vi "Auton File Loader.vi"() -> ()   [LabVIEW 2017]
uses:
  Common Code/Auton File Lists.ctl
  Robot Global Data.vi
panel:
  in  "Auton File Lists":T1
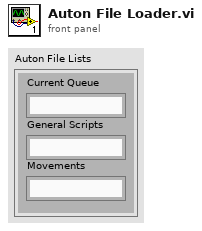
[diagram p1: front panel]
types:
  T1 = typedef "Auton File Lists.ctl" = cluster{"Current Queue":string, "General Scripts":string, "Movements":string}
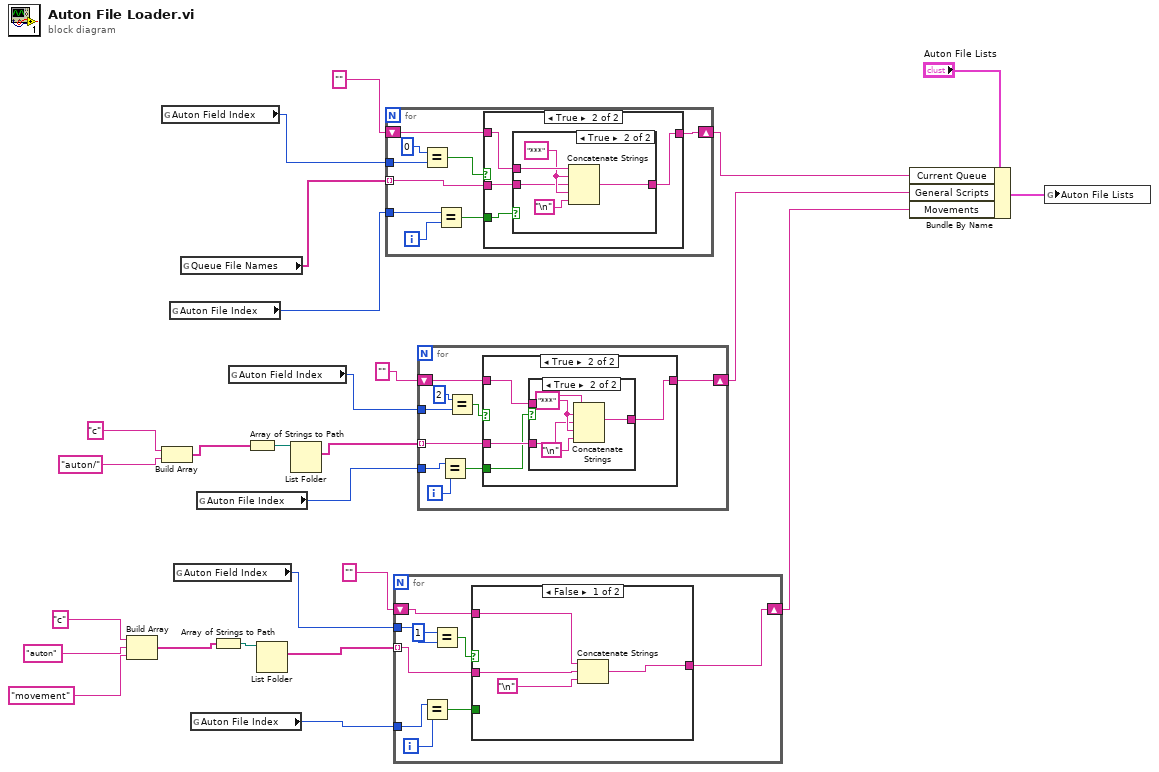
[diagram p0: block diagram]
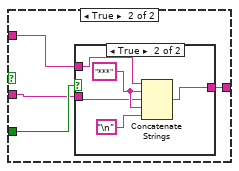
[diagram p2: hidden frame]
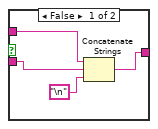
[diagram p3: hidden frame]
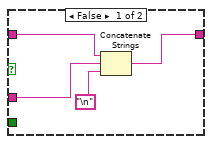
[diagram p4: hidden frame]
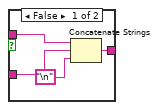
[diagram p5: hidden frame]
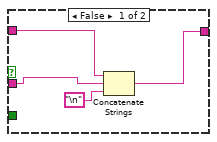
[diagram p6: hidden frame]
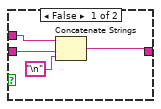
[diagram p7: hidden frame]
diagram:
  n1 = Build Array("c", "auton", "movement") -> (w5:string[])
  n2 = global read "Robot Global Data.vi" "Auton Field Index"() -> (w22:i32)
  n3 = Build Array("c", "auton/") -> (w15:string[])
  n4 = global read "Robot Global Data.vi" "Auton File Index"() -> (w19:i32)
  n5 = global read "Robot Global Data.vi" "Auton Field Index"() -> (w9:i32)
  n6 = global read "Robot Global Data.vi" "Queue File Names"() -> (w20:string[])
  n7 = global read "Robot Global Data.vi" "Auton File Index"() -> (w10:i32)
  n8 = global read "Robot Global Data.vi" "Auton File Index"() -> (w13:i32)
  n9 = Array of Strings to Path(0:w5) -> (2:w6:path)  [unwired: 1 in]
  n10 = global read "Robot Global Data.vi" "Auton Field Index"() -> (w1:i32)
  n11 = Array of Strings to Path(0:w15) -> (2:w16:path)  [unwired: 1 in]
  n12 = List Folder(path=w6) -> (filenames=w3:string[])  [unwired: 3 in, 3 out]
  n13 = List Folder(path=w16) -> (filenames=w14:string[])  [unwired: 3 in, 3 out]
  n14 = for {
    tunnel: w20 -> [w30] mode=indexing
    shift-right: [w29] -> w26
    shift-left: "" -> [w31]
    tunnel: w22 -> [w28]
    tunnel: w19 -> [w27]
    i -> [w33]
    n15 = Equal?(x=0, y=w28) -> (x = y?=w34:bool)
    n16 = Equal?(x=w27, y=w33) -> (x = y?=w32:bool)
    n17 = case shown="True" w34 {
      tunnel: w32 -> [_ w43]
      tunnel: w31 -> [w39 w42]
      tunnel: w30 -> [w36 w41]
      tunnel: [w37 w40] -> w29
      frame False {
        n18 = Concatenate Strings(w39, w36, "\n") -> (w37:string)
      }
      frame True {
        n19 = case shown="True" w43 {
          tunnel: w42 -> [w47 w52]
          tunnel: w41 -> [w44 w48]
          tunnel: [w45 w49] -> w40
          frame False {
            n20 = Concatenate Strings(w47, w44, "\n") -> (w45:string)
          }
          frame True {
            w51 = "***"
            n21 = Concatenate Strings(w52, w51, w48, w51, "\n") -> (w49:string)
          }
        }
      }
    }
  }
  n22 = for {
    shift-right: [w53] -> w24
    shift-left: "" -> [w61]
    tunnel: w3 -> [w60] mode=indexing
    tunnel: w9 -> [w58]
    tunnel: w10 -> [w56]
    i -> [w55]
    n23 = Equal?(x=w56, y=w55) -> (x = y?=w54:bool)
    n24 = Equal?(x=1, y=w58) -> (x = y?=w57:bool)
    n25 = case shown="False" w57 {
      tunnel: w61 -> [w65 w69]
      tunnel: w60 -> [w64 w67]
      tunnel: w54 -> [_ w68]
      tunnel: [w62 w66] -> w53
      frame False {
        n26 = Concatenate Strings(w65, w64, "\n") -> (w62:string)
      }
      frame True {
        n27 = case shown="True" w68 {
          tunnel: w69 -> [w72 w75]
          tunnel: w67 -> [w71 w76]
          tunnel: [w73 w74] -> w66
          frame False {
            n28 = Concatenate Strings(w72, w71, "\n") -> (w73:string)
          }
          frame True {
            w78 = "***"
            n29 = Concatenate Strings(w75, w78, w76, w78, "\n") -> (w74:string)
          }
        }
      }
    }
  }
  n30 = for {
    shift-right: [w85] -> w23
    shift-left: "" -> [w87]
    tunnel: w14 -> [w86] mode=indexing
    tunnel: w13 -> [w83]
    tunnel: w1 -> [w79]
    i -> [w84]
    n31 = Equal?(x=w83, y=w84) -> (x = y?=w80:bool)
    n32 = Equal?(x=2, y=w79) -> (x = y?=w81:bool)
    n33 = case shown="True" w81 {
      tunnel: w87 -> [w91 w95]
      tunnel: w86 -> [w90 w94]
      tunnel: [w88 w93] -> w85
      tunnel: w80 -> [_ w92]
      frame False {
        n34 = Concatenate Strings(w91, w90, "\n") -> (w88:string)
      }
      frame True {
        n35 = case shown="True" w92 {
          tunnel: w95 -> [w99 w102]
          tunnel: w94 -> [w98 w101]
          tunnel: [w96 w104] -> w93
          frame False {
            n36 = Concatenate Strings(w99, w98, "\n") -> (w96:string)
          }
          frame True {
            w103 = "***"
            n37 = Concatenate Strings(w102, w103, w101, w103, "\n") -> (w104:string)
          }
        }
      }
    }
  }
  n38 = Bundle By Name(cluster="Auton File Lists", "Current Queue"=w26, "General Scripts"=w23, "Movements"=w24) -> (w12:T1)
  n39 = global write "Robot Global Data.vi" "Auton File Lists"(w12) -> ()
